vi "FTW-File-IsRelative.vi"(1 "Filepath":path) -> (0 "Relative?":bool)   [LabVIEW 2012]
panel:
  # "Inputs"
  # "Outputs"
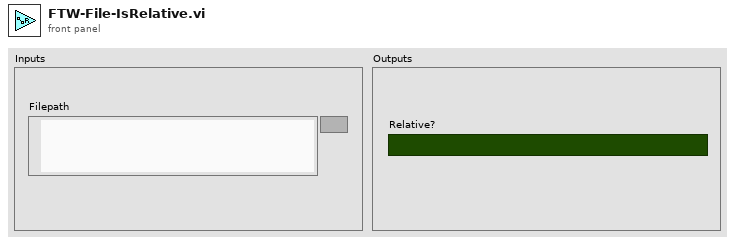
[diagram p1: front panel]
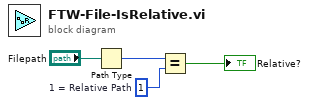
[diagram p0: block diagram]
diagram:
  w1 = i16 1  # 1 = Relative Path
  n1 = Path Type(1:"Filepath") -> (0:w4:i16)
  n2 = Equal?(x=w4, y=w1) -> (x = y?=→"Relative?":bool)
